vi "Read Message.vi"(6 "error in":errorcluster, 8 "timeout ms (5000)":i32=5000, 9 "RawSocket Handler in":refnum<class "RawSocket Handler.lvclass">) -> (0 "error out":errorcluster, 1 "Message data":string, 2 "Message Type":T1, 3 "RawSocket Handler out":refnum<class "RawSocket Handler.lvclass">)   [LabVIEW 2020, in "wamplv.lvlib" / "RawSocket Handler.lvclass"]
uses:
  RawSocket Handler.lvclass
  Message Type.ctl
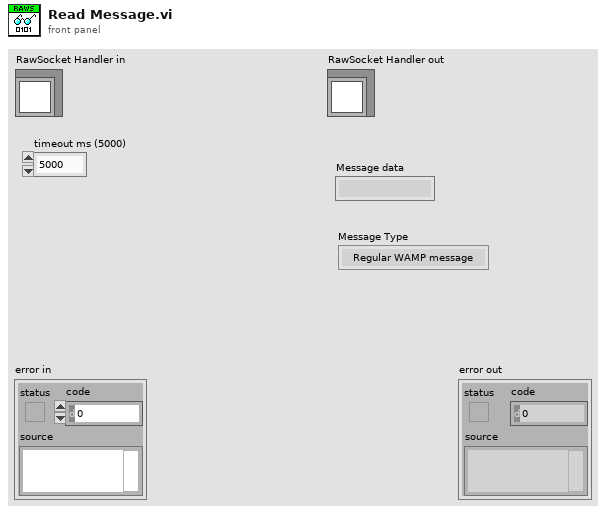
[diagram p1: front panel]
types:
  T1 = typedef "wamplv.lvlib/RawSocket Handler.lvclass/Message Type.ctl" = enum16{"Regular WAMP message", "PING", "PONG"}
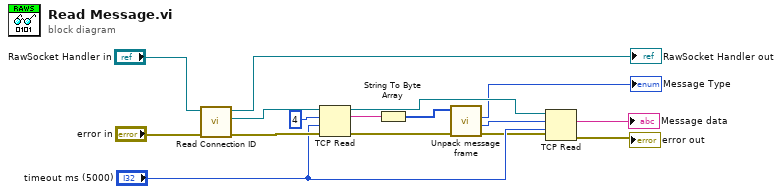
[diagram p0: block diagram]
diagram:
  n1 = call-dynamic "Read Connection ID.vi"("error in (no error)"="error in", "RawSocket Handler in"="RawSocket Handler in") -> ("error out"=w13:errorcluster, "Connection ID"=w12:refnum<k5>, "RawSocket Handler out"=→"RawSocket Handler out":refnum<class "RawSocket Handler.lvclass">)  [unwired: 7 in]
  n2 = TCP Read(connection ID=w12, bytes to read=4, error in (no error)=w13, 9:"timeout ms (5000)") -> (connection ID out=w10:refnum<k5>, data out=w8:string, error out=w9:errorcluster)  [unwired: 1 in]
  n3 = String To Byte Array(string=w8) -> (unsigned byte array=w7:u8[])
  n4 = call "Unpack message frame.vi"("error in"=w9, "Message frame"=w7) -> ("error IO"=w5:errorcluster, "Size (bytes)"=w4:i32, "Message Type"=→"Message Type":T1)  [unwired: 7 in]
  n5 = TCP Read(connection ID=w10, bytes to read=w4, error in (no error)=w5, 9:"timeout ms (5000)") -> (data out=→"Message data":string, error out=→"error out":errorcluster)  [unwired: 1 in, 1 out]
